vi "writeToXML.vi"(8 "error in (no error)":errorcluster, 10 "ClassLabel":string, 11 "ScienceTargetClearOffset in":refnum<class "ScienceTargetClearOffset.lvclass">) -> (0 "error out":errorcluster, 2 "XML out":string, 3 "ScienceTargetClearOffset out":refnum<class "ScienceTargetClearOffset.lvclass">)   [LabVIEW 2022 SP3, in "TCSDataDefinitions.lvlib" / "TCSCommand.lvlib" / "OffsetCommands.lvlib" / "ScienceTargetClearOffset.lvclass"]
uses:
  ScienceTargetClearOffset.lvclass
  ClearOffset/ClearOffset.lvclass
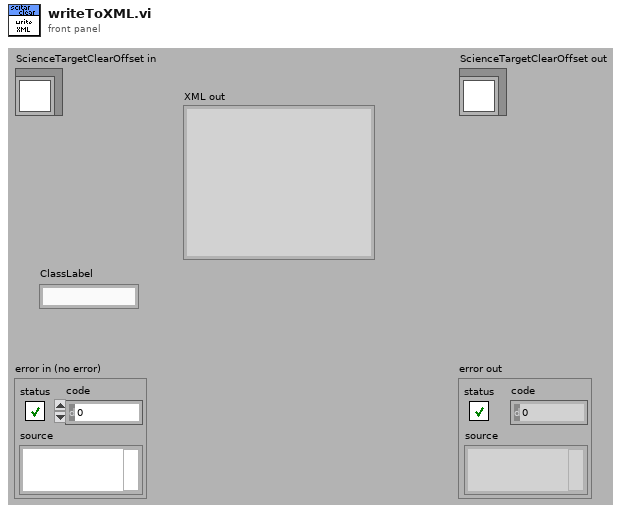
[diagram p1: front panel]
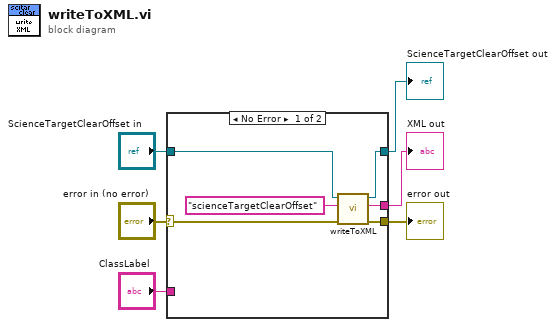
[diagram p0: block diagram]
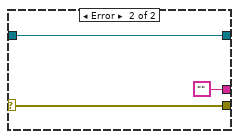
[diagram p2: hidden frame]
diagram:
  n1 = case shown="No Error" "error in (no error)" {
    selector: "error in (no error)" -> [w10 w15]
    tunnel: [w9 w15] -> w5
    tunnel: [w11 w14] -> w3
    tunnel: "ScienceTargetClearOffset in" -> [w12 w14]
    tunnel: [w8 ""] -> w2
    tunnel: "ClassLabel" -> [_ _]
    frame No Error {
      n2 = call-parent "writeToXML.vi"("error in (no error)"=w10, "ClassLabel"="scienceTargetClearOffset", "ClearOffset in"=w12) -> ("error out"=w9:errorcluster, "XML out"=w8:string, "ClearOffset out"=w11:refnum<class "ScienceTargetClearOffset.lvclass">)  [unwired: 6 in]
    }
    frame Error {
    }
  }
  "error out" <- w5
  "ScienceTargetClearOffset out" <- w3
  "XML out" <- w2
